vi "GetLoggerInformation.vi"(8 "error in (no error)":errorcluster, 11 "Logger in":refnum<class "Logger.lvclass">) -> (0 "error out":errorcluster, 2 "Logger information":T1={"Log File Path"="", "Verbosity"=enum."Default", "Append to log file?"=FALSE}, 3 "Logger out":refnum<class "Logger.lvclass">)   [LabVIEW 2014, in "Logger.lvclass"]
uses:
  Logger.lvclass
  LoggerCore.ctl
  Logger.lvclass/Logger.ctl
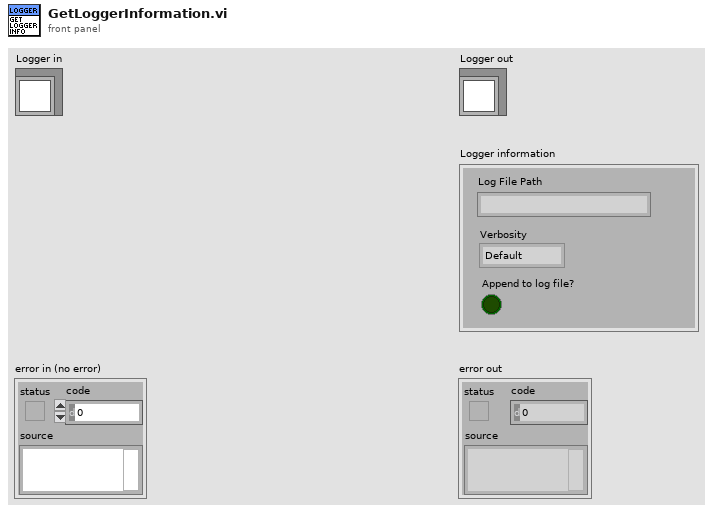
[diagram p1: front panel]
types:
  T1 = typedef "Logger.lvclass/LoggerCore.ctl" = cluster{"Log File Path":string, "Verbosity":enum16{"Minimal", "Default", "Detailed", "Diagnostic"}, "Append to log file?":bool}
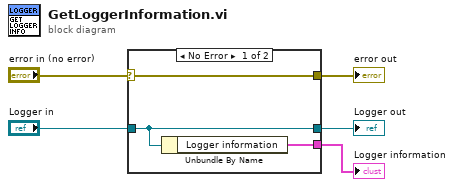
[diagram p0: block diagram]
diagram:
  n1 = case shown="No Error" "error in (no error)" {
    selector: "error in (no error)" -> [w8 w9]
    tunnel: [w8 w9] -> w4
    tunnel: [w7 w10] -> w2
    tunnel: "Logger in" -> [w7 w10]
    tunnel: [w6 _] -> w1
    frame No Error {
      n2 = Unbundle By Name(w7) -> ("Logger information"=w6:T1)
    }
    frame Error {
    }
  }
  "error out" <- w4
  "Logger out" <- w2
  "Logger information" <- w1
